vi "Launch.vi"(8 "error in (no error)":errorcluster, 10 "index":i32, 11 "User Interface in":refnum<class "User Interface.lvclass">) -> (0 "error out":errorcluster, 2 "active ref":refnum<vi>, 3 "User Interface out":refnum<class "User Interface.lvclass">)   [LabVIEW 2017, in "DSF Core.lvlib" / "User Interface.lvclass"]
uses:
  User Interface.lvclass
  Configuration/Configuration.lvclass
  User Interface Events/User Interface Events.lvclass
  User Interface.lvclass/User Interface.ctl
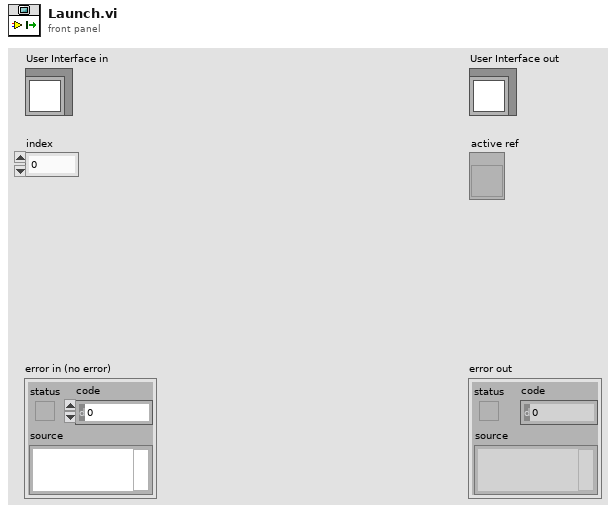
[diagram p1: front panel]
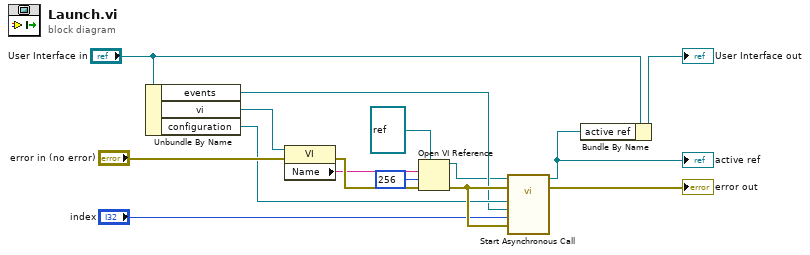
[diagram p0: block diagram]
diagram:
  n1 = Unbundle By Name("User Interface in") -> ("events"=w4:refnum<class "User Interface Events.lvclass">, "vi"=w2:refnum<vi>, "configuration"=w5:refnum<class "Configuration.lvclass">)
  n2 = property class="VI"(reference=w2, error in="error in (no error)") -> (error out=w12:errorcluster, "Name"=w10:string)  [unwired: 1 out]
  n3 = Open VI Reference(type specifier VI Refnum (for type only)=refnum<vi> refnum, vi path=w10, options=256, error in (no error)=w12) -> (vi reference=w1:refnum<vi>, error out=w14:errorcluster)  [unwired: 2 in]
  n4 = call-by-ref "Start Asynchronous Call"(reference=w1, error in=w14, 8:"error in (no error)"=w14, "index"="index", "User Interface Events"=w4, "Configuration in"=w5) -> (reference out=w7:refnum<vi>, error out=→"error out":errorcluster)  [unwired: 6 in, 2 out]
  "active ref" <- w7
  n5 = Bundle By Name(cluster="User Interface in", "active ref"=w7) -> (→"User Interface out":refnum<class "User Interface.lvclass">)
